vi "Switch Child Symbol.vi"(8 "Symbols":i32[](array[numeric]), 10 "Parent Tag":string, 11 "Tree in":refnum<class "Tree.lvclass">) -> (3 "Tree out":refnum<class "Tree.lvclass">)   [LabVIEW 2022 SP3, in "Tree.lvclass"]
uses:
  Tree.lvclass
  Tree.lvclass/Tree.ctl
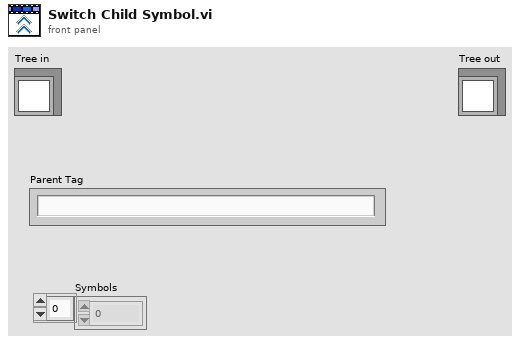
[diagram p1: front panel]
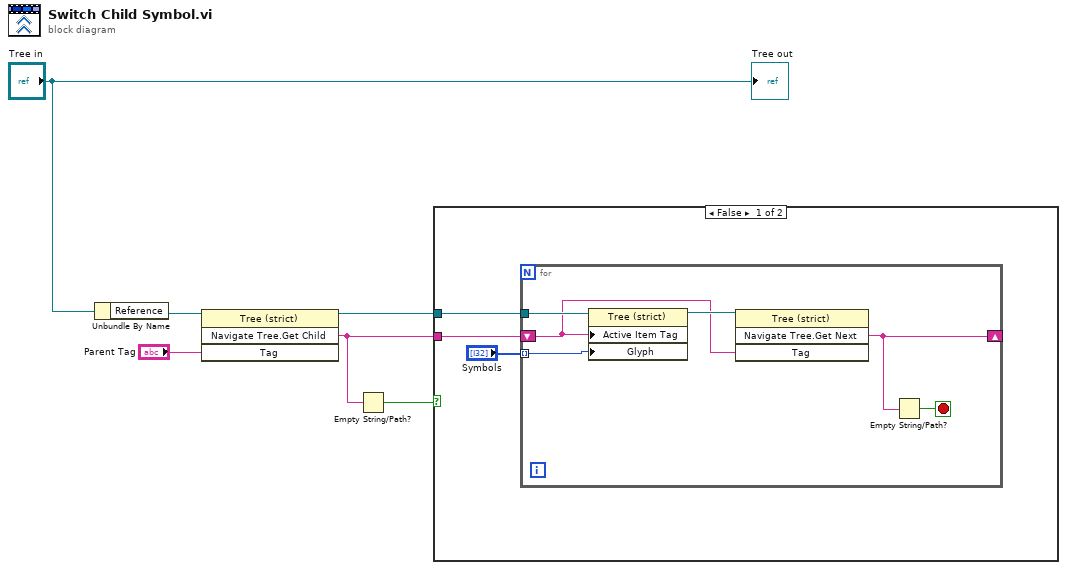
[diagram p0: block diagram]
diagram:
  n1 = Unbundle By Name("Tree in") -> ("Reference"=w1:refnum<vi>)
  n2 = invoke class="Tree (strict)" method="Navigate Tree.Get Child"(reference=w1, "Tag"="Parent Tag") -> (reference out=w5:refnum<vi>, "Navigate Tree:Get Child"=w3:string)  [unwired: 2 in, 2 out]
  n3 = Empty String/Path?(string/path=w3) -> (empty?=w2:bool)
  n4 = case shown="False" w2 {
    tunnel: w5 -> [w9 _]
    tunnel: w3 -> [w7 _]
    frame False {
      n5 = for {
        shift-right: [w12] -> _
        shift-left: w7 -> [w13]
        tunnel: "Symbols" -> [w10] mode=indexing
        tunnel: w9 -> [w15]
        stop <- w11 stop-if-true
        n6 = property class="Tree (strict)"(reference=w15, "Active Item Tag"=w13, "Glyph"=w10) -> (reference out=w14:refnum<vi>)  [unwired: 1 in, 1 out]
        n7 = invoke class="Tree (strict)" method="Navigate Tree.Get Next"(reference=w14, "Tag"=w13) -> ("Navigate Tree:Get Next Item"=w12:string)  [unwired: 2 in, 3 out]
        n8 = Empty String/Path?(string/path=w12) -> (empty?=w11:bool)
      }
    }
    frame True {
    }
  }
  "Tree out" <- "Tree in"
